vi "Counter.vi"(3 "Reset":bool, 4 "TimerConfig":T3, 5 "AnalogTriggers":T2[](array[typedef])=[{"InHysteresis"=FALSE, "OverLimit"=FALSE, "Rising"=FALSE, "Falling"=FALSE}, {"InHysteresis"=FALSE, "OverLimit"=FALSE, "Rising"=FALSE, "Falling"=FALSE}, {"InHysteresis"=FALSE, "OverLimit"=FALSE, "Rising"=FALSE, "Falling"=FALSE}, {"InHysteresis"=FALSE, "OverLimit"=FALSE, "Rising"=FALSE, "Falling"=FALSE}, {"InHysteresis"=FALSE, "OverLimit"=FALSE, "Rising"=FALSE, "Falling"=FALSE}, {"InHysteresis"=FALSE, "OverLimit"=FALSE, "Rising"=FALSE, "Falling"=FALSE}, {"InHysteresis"=FALSE, "OverLimit"=FALSE, "Rising"=FALSE, "Falling"=FALSE}, {"InHysteresis"=FALSE, "OverLimit"=FALSE, "Rising"=FALSE, "Falling"=FALSE}], 6 "DigitalInputs":bool[](array[boolean])=[FALSE, FALSE, FALSE, FALSE, FALSE, FALSE, FALSE, FALSE, FALSE, FALSE, FALSE, FALSE, FALSE, FALSE, FALSE, FALSE, FALSE, FALSE, FALSE, FALSE, FALSE, FALSE, FALSE, FALSE, FALSE, FALSE, FALSE, FALSE, FALSE, FALSE, FALSE, FALSE], 7 "Config":T4) -> (0 "TimerOutput":T1, 1 "Output":T6)   [LabVIEW 2019]
uses:
  Controls/Counter_Output.ctl
  Controls/Counter_Config.ctl
  Helpers/Source.ctl
  Controls/TimerConfig.ctl
  Helpers/AnalogTriggerOutput.ctl
  Helpers/TimerOutput.ctl
  <vilib>/rvi/Emulation/niFpgaSctlEmulationGetInTimedLoop.vi
  <vilib>/rvi/Emulation/niFpgaProcessEmulError.vi
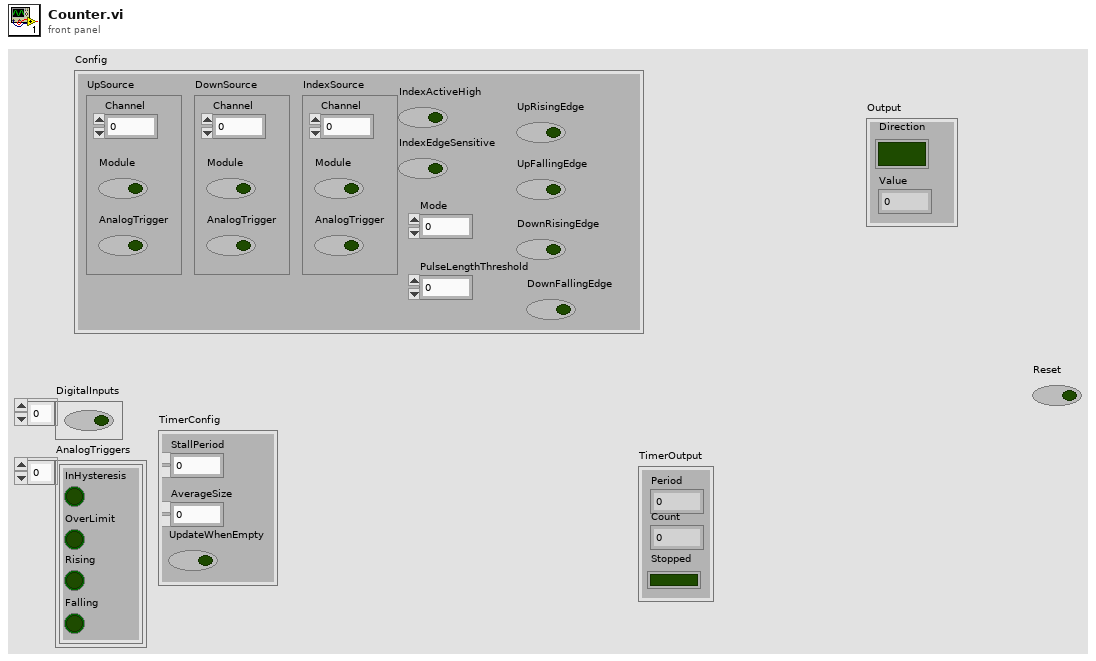
[diagram p1: front panel]
types:
  T1 = typedef "TimerOutput.ctl" = cluster{"Period":fxp<+,24,25>, "Count":i16, "Stopped":bool}
  T2 = typedef "AnalogTriggerOutput.ctl" = cluster{"InHysteresis":bool, "OverLimit":bool, "Rising":bool, "Falling":bool}
  T3 = typedef "TimerConfig.ctl" = cluster{"StallPeriod":fxp<+,24,24>, "AverageSize":fxp<+,7,7>, "UpdateWhenEmpty":bool}
  T4 = typedef "Counter_Config.ctl" = cluster{"UpSource":T5, "DownSource":T5, "IndexSource":T5, "IndexActiveHigh":bool, "IndexEdgeSensitive":bool, "UpRisingEdge":bool, "UpFallingEdge":bool, "DownRisingEdge":bool, "DownFallingEdge":bool, "Mode":fxp<+,2,2>, "PulseLengthThreshold":fxp<+,6,14>}
  T5 = typedef "Source.ctl" = cluster{"Channel":fxp<+,4,4>, "Module":bool, "AnalogTrigger":bool}
  T6 = typedef "Counter_Output.ctl" = cluster{"Direction":bool, "Value":fxp<+/-,31,31>}
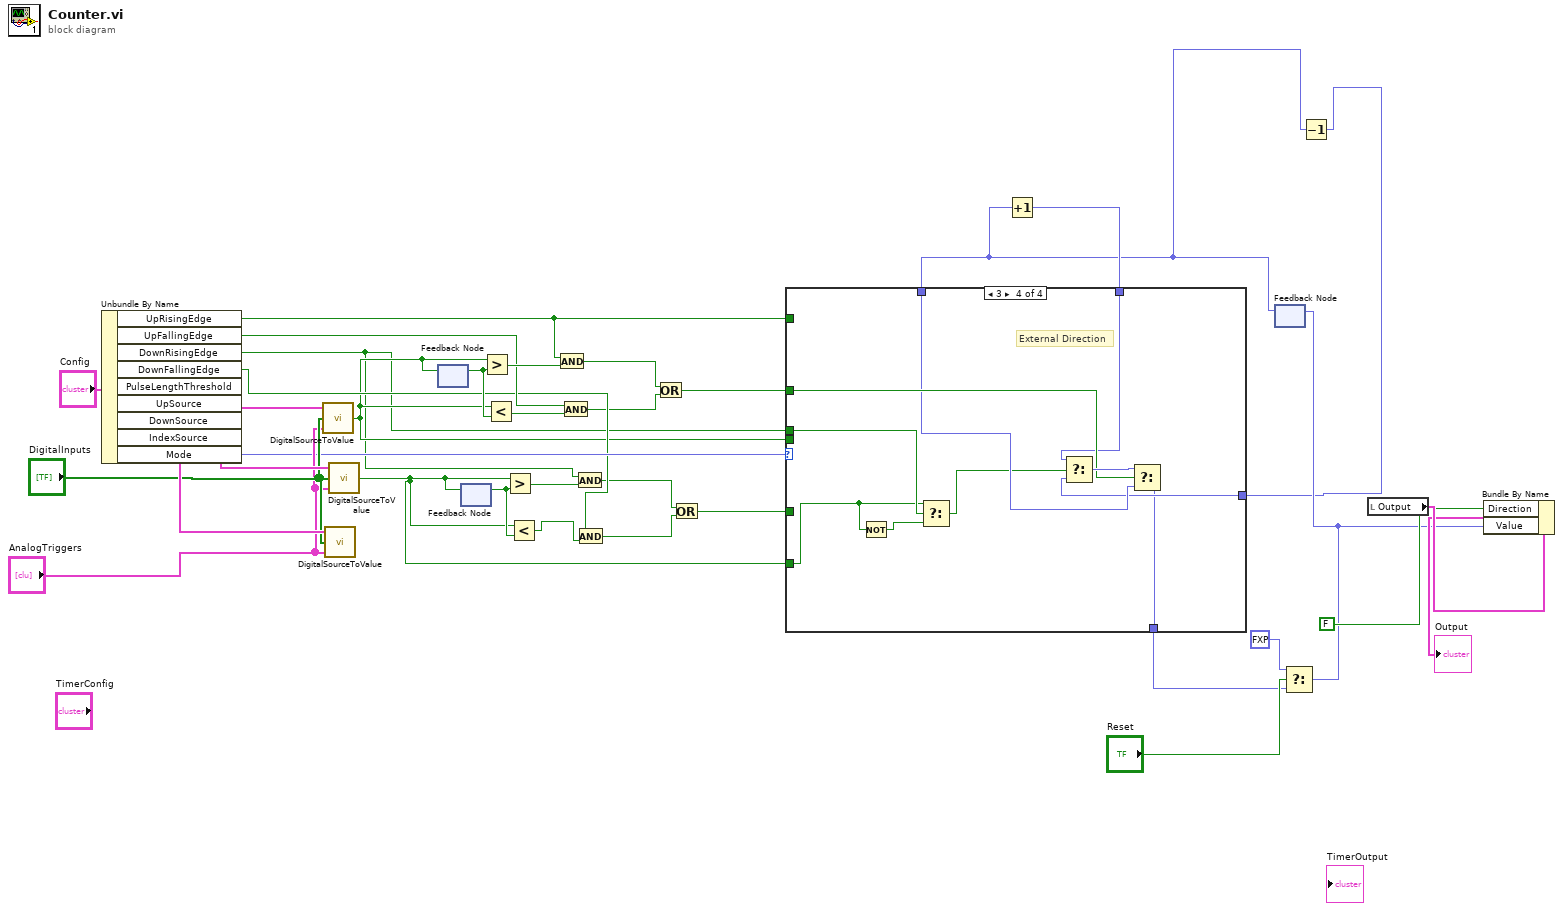
[diagram p0: block diagram]
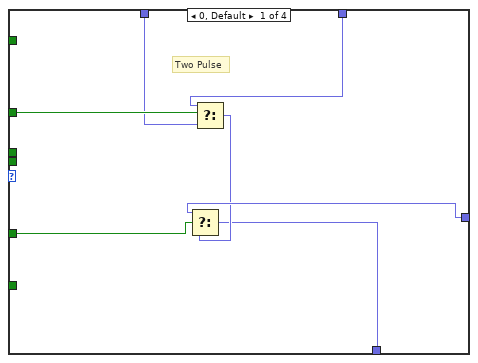
[diagram p2: hidden frame]
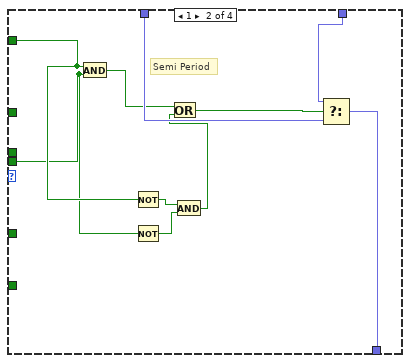
[diagram p3: hidden frame]
diagram:
  n1 = Unbundle By Name("Config") -> ("UpRisingEdge"=w6:bool, "UpFallingEdge"=w18:bool, "DownRisingEdge"=w4:bool, "DownFallingEdge"=w15:bool, "UpSource"=w34:T5, "DownSource"=w33:T5, "IndexSource"=w32:T5, "Mode"=w26:fxp<+,2,2>)  [unwired: 1 out]
  n2 = call "DigitalSourceToValue.vi"("AnalogTriggers"="AnalogTriggers", "DigitalInputs"="DigitalInputs", "Source"=w34) -> ("Value"=w5:bool)
  n3 = call "DigitalSourceToValue.vi"("AnalogTriggers"="AnalogTriggers", "DigitalInputs"="DigitalInputs", "Source"=w32) -> ()  [unwired: 1 out]
  n4 = call "DigitalSourceToValue.vi"("AnalogTriggers"="AnalogTriggers", "DigitalInputs"="DigitalInputs", "Source"=w33) -> ("Value"=w10:bool)
  n5 = feedback-in #1(w5) -> ()
  n6 = feedback #1() -> (w25:bool)  [unwired: 1 in]
  n7 = feedback #2() -> (w24:bool)  [unwired: 1 in]
  n8 = feedback-in #2(w10) -> ()
  n9 = Greater?(x=w5, y=w25) -> (0:w20:bool)
  n10 = Less?(x=w5, y=w25) -> (x < y?=w19:bool)
  n11 = Greater?(x=w10, y=w24) -> (0:w17:bool)
  n12 = Less?(x=w10, y=w24) -> (x < y?=w16:bool)
  n13 = And(x=w6, y=w20) -> (x .and. y?=w14:bool)
  n14 = And(x=w18, y=w19) -> (x .and. y?=w13:bool)
  n15 = And(x=w4, y=w17) -> (x .and. y?=w9:bool)
  n16 = And(x=w15, y=w16) -> (x .and. y?=w8:bool)
  n17 = Or(x=w14, y=w13) -> (x .or. y?=w12:bool)
  n18 = Or(x=w9, y=w8) -> (x .or. y?=w7:bool)
  n19 = feedback #3() -> (w2:fxp<+/-,31,31>)  [unwired: 1 in]
  n20 = Increment(x=w2) -> (x+1=w3:fxp<+/-,31,31>)
  n21 = Decrement(x=w2) -> (x-1=w1:fxp<+/-,31,31>)
  n22 = case shown="3" w26 {
    tunnel: w2 -> [w38 w52 w53 w61]
    tunnel: w12 -> [w42 _ _ w62]
    tunnel: w3 -> [w41 w46 _ w60]
    tunnel: w1 -> [w39 _ _ w59]
    tunnel: [w36 w43 w53 w58] -> w11
    tunnel: w10 -> [_ _ _ w56]
    tunnel: w7 -> [w40 _ _ _]
    tunnel: w6 -> [_ w45 _ _]
    tunnel: w5 -> [_ w44 _ _]
    tunnel: w4 -> [_ _ _ w57]
    frame 0, Default {
      # "Two Pulse"
      n23 = Select(t=w41, s=w42, f=w38) -> (s? t:f=w37:fxp<+/-,31,31>)
      n24 = Select(t=w39, s=w40, f=w37) -> (s? t:f=w36:fxp<+/-,31,31>)
    }
    frame 1 {
      # "Semi Period"
      n25 = And(x=w45, y=w44) -> (x .and. y?=w51:bool)
      n26 = Not(x=w45) -> (.not. x?=w50:bool)
      n27 = Not(x=w44) -> (.not. x?=w49:bool)
      n28 = And(x=w50, y=w49) -> (x .and. y?=w48:bool)
      n29 = Or(x=w51, y=w48) -> (x .or. y?=w47:bool)
      n30 = Select(t=w46, s=w47, f=w52) -> (s? t:f=w43:fxp<+/-,31,31>)
    }
    frame 2 {
      # "Pulse Length"
    }
    frame 3 {
      # "External Direction"
      n31 = Not(x=w56) -> (.not. x?=w55:bool)
      n32 = Select(t=w56, s=w57, f=w55) -> (s? t:f=w54:bool)
      n33 = Select(t=w60, s=w54, f=w59) -> (s? t:f=w63:fxp<+/-,31,31>)
      n34 = Select(t=w63, s=w62, f=w61) -> (s? t:f=w58:fxp<+/-,31,31>)
    }
  }
  n35 = Select(t=fxp<+/-,31,31> 0.0 ("Value"), s="Reset", f=w11) -> (s? t:f=w21:fxp<+/-,31,31>)
  n36 = feedback-in #3(w21) -> ()
  n37 = local read "Output"() -> (w30:T6)
  n38 = Bundle By Name(cluster=w30, "Direction"=FALSE, "Value"=w21) -> (→"Output":T6)
